vi "多态-带索引冒泡排序.vi"   [LabVIEW 2013]
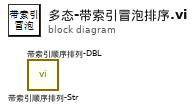
[diagram p0: block diagram]
diagram:
  n1 = call "带索引顺序排列-Str.vi"() -> ()  [unwired: 10 in, 2 out]
  n2 = call "带索引顺序排列-DBL.vi"() -> ()  [unwired: 10 in, 2 out]
